vi "Set Standard.vi"(8 "error in (no error)":errorcluster, 10 "802.11 Standard":T1, 11 "niDTS WLAN Dut in":refnum<class "niDTS WLAN Dut.lvclass">) -> (0 "error out":errorcluster, 3 "niDTS WLAN Dut out":refnum<class "niDTS WLAN Dut.lvclass">)   [LabVIEW 2015, in "niDTS WLAN.lvlib" / "niDTS WLAN Dut.lvclass"]
doc: "Sets the 802.11 Standard to one of \n* 802.11 b DSSS\n* 802.11 ag OFDM\n* 802.11 n HT\n* 802.11 ac VHT\n\nCallbacks:\n* Update Type\n* Update Payload Length"
uses:
  niDTS WLAN Dut.lvclass
  Includes/niDTS WLAN INC Standard.ctl
  niDTS WLAN Dut.lvclass/niDTS WLAN Dut.ctl
  niDTS WLAN.lvlib
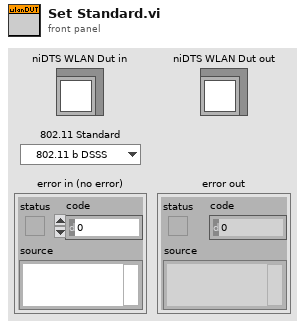
[diagram p1: front panel]
types:
  T1 = typedef "niDTS WLAN.lvlib/niDTS WLAN INC Standard.ctl" = enum16{"802.11 b DSSS", "802.11 a/g OFDM", "802.11 n HT", "802.11 ac VHT"}
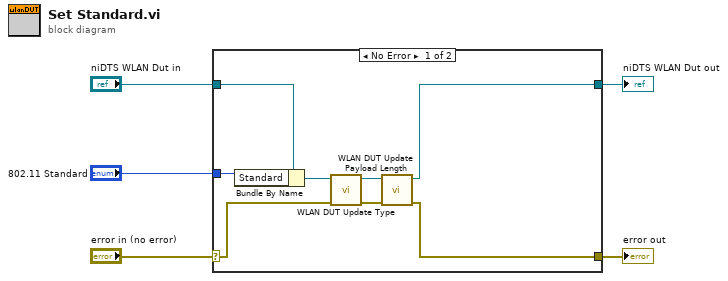
[diagram p0: block diagram]
diagram:
  n1 = case shown="No Error" "error in (no error)" {
    selector: "error in (no error)" -> [w10 w14]
    tunnel: [w8 w14] -> w4
    tunnel: [w6 w15] -> w2
    tunnel: "niDTS WLAN Dut in" -> [w13 w15]
    tunnel: "802.11 Standard" -> [w12 _]
    frame No Error {
      n2 = Bundle By Name(cluster=w13, "Standard"=w12) -> (w11:refnum<class "niDTS WLAN Dut.lvclass">)
      n3 = call-dynamic "WLAN DUT Update Type.vi"("error in (no error)"=w10, "niDTS WLAN DUT in"=w11) -> ("error out"=w9:errorcluster, "niDTS WLAN DUT out"=w7:refnum<class "niDTS WLAN Dut.lvclass">)  [unwired: 8 in]
      n4 = call-dynamic "WLAN DUT Update Payload Length.vi"("error in (no error)"=w9, "niDTS WLAN DUT in"=w7) -> ("error out"=w8:errorcluster, "niDTS WLAN DUT out"=w6:refnum<class "niDTS WLAN Dut.lvclass">)  [unwired: 8 in]
    }
    frame Error {
    }
  }
  "error out" <- w4
  "niDTS WLAN Dut out" <- w2
